vi "Time Estimate.vi"(8 "error in (no error)":errorcluster, 10 "Points":dbl, 11 "Photon Counter with LCD Reader in":refnum<class "Photon Counter with LCD Reader.lvclass">) -> (0 "error out":errorcluster, 2 "time":dbl[unit], 3 "Photon Counter with LCD Reader out":refnum<class "Photon Counter with LCD Reader.lvclass">)   [LabVIEW 2023, in "Photon Counter with LCD Reader.lvclass"]
uses:
  Photon Counter with LCD Reader.lvclass
  Photon Counter with LCD Reader.lvclass/Photon Counter with LCD Reader.ctl
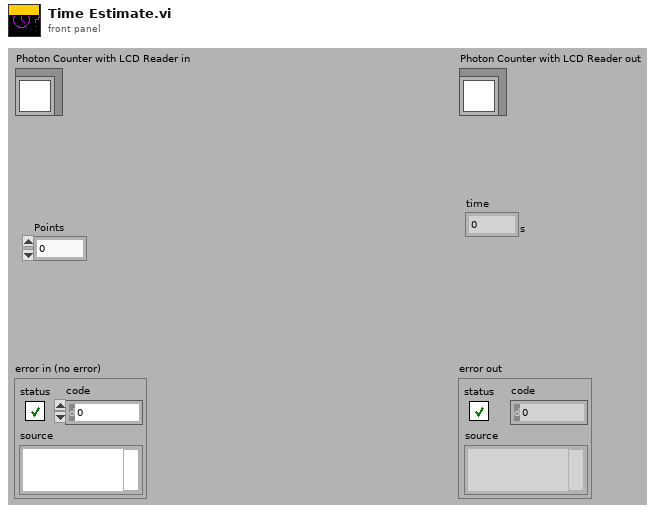
[diagram p1: front panel]
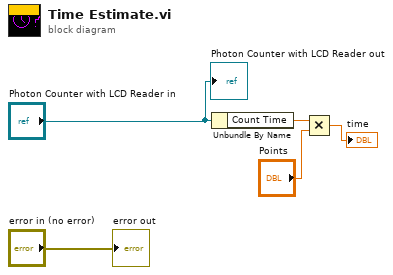
[diagram p0: block diagram]
diagram:
  n1 = Unbundle By Name("Photon Counter with LCD Reader in") -> ("Count Time"=w3:dbl[unit])
  n2 = Multiply(x=w3, y="Points") -> (x*y=→"time":dbl[unit])
  "error out" <- "error in (no error)"
  "Photon Counter with LCD Reader out" <- "Photon Counter with LCD Reader in"
